vi "LV Mass Compile.vi"   [LabVIEW 2016, in "Script.lvlib"]
uses:
  Script.lvlib
  <vilib>/Wiresmith Technology/G CLI/Argument Parser/Option Class/Option Configuration.ctl
  <vilib>/Wiresmith Technology/G CLI/Argument Parser/Option Class/Argument Type.ctl
  <vilib>/Wiresmith Technology/G CLI/CLI Class/CLI.lvclass
  <vilib>/Wiresmith Technology/G CLI/Argument Parser/Option Class/Option.lvclass
  <vilib>/Wiresmith Technology/G CLI/Argument Parser/Option Set Class/Option Set.lvclass
types:
  T1 = typedef "Option Parser.lvlib/Option.lvclass/Option Configuration.ctl" = cluster{"Option Type":T2, "Option Labels":string[], "Key":string, "Description":string, "Required":bool, "Default Value":string}
  T2 = typedef "Option Parser.lvlib/Option.lvclass/Argument Type.ctl" = enum16{"flag", "value"}
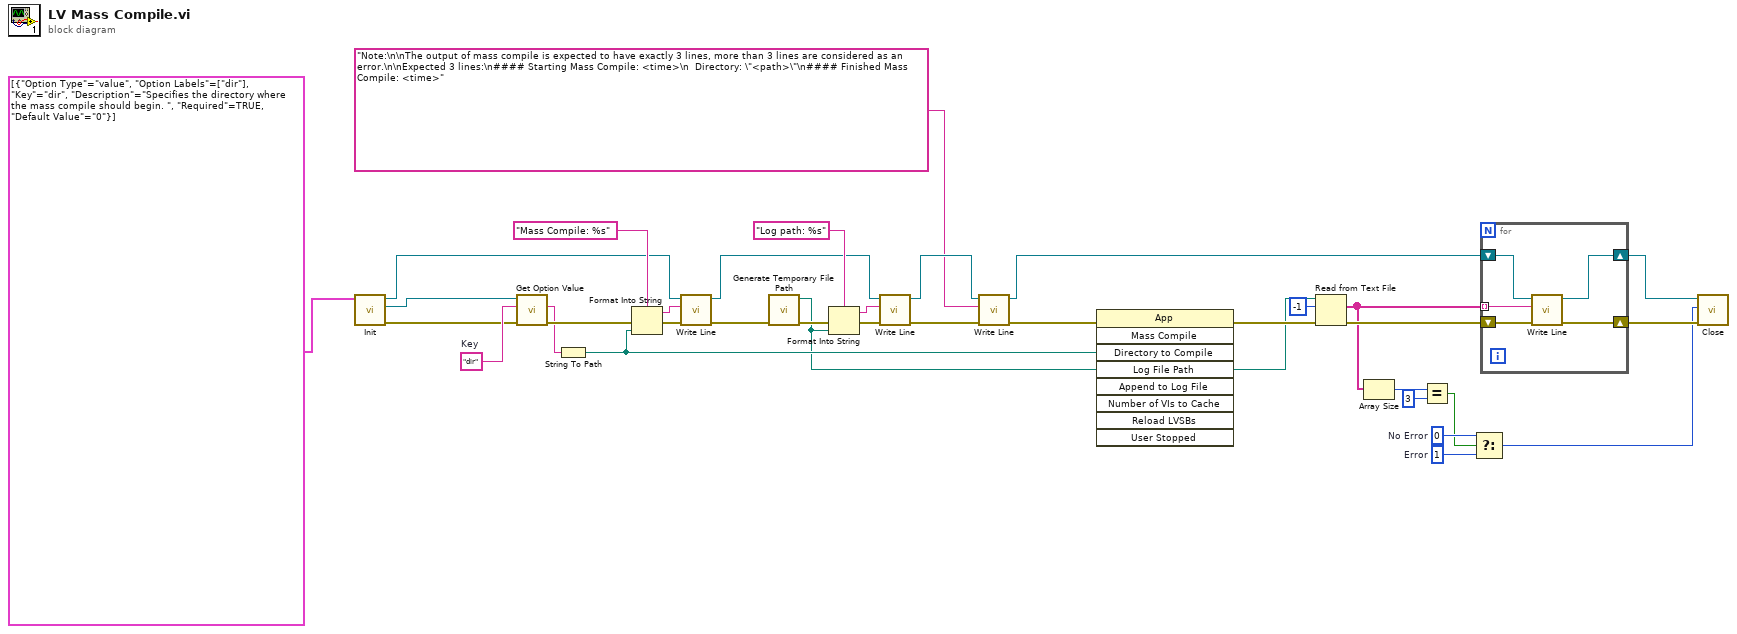
[diagram p0: block diagram]
diagram:
  w10 = 1  # Error
  w11 = 0  # No Error
  w35 = "dir"  # Key
  n1 = call "Init.vi"("Options"=T1[] [{"Option Type"=enum."value", "Option Labels"=["dir"], "Key"="dir", "Description"="Specifies the directory where the mass compile should begin. ", "Required"=TRUE, "Default Value"="0"}]) -> ("error out"=w18:errorcluster, "Option Set out"=w16:refnum<class "Option Set.lvclass">, "CLI out"=w17:refnum<class "CLI.lvclass">)  [unwired: 8 in]
  n2 = call <vilib>:"Get Option Value.vi"("error in (no error)"=w18, "Option Key"=w35, "Option Set in"=w16) -> ("error out"=w30:errorcluster, "Value"=w26:string)  [unwired: 5 in, 2 out]
  n3 = String To Path(string=w26) -> (path=w25:path)
  n4 = Format Into String(format string="Mass Compile: %s", error in=w30, w25) -> (resulting string=w24:string, error out=w29:errorcluster)  [unwired: 1 in]
  n5 = call <vilib>:"Write Line.vi"("error in (no error)"=w29, "Text to Write"=w24, "CLI in"=w17) -> ("error out"=w34:errorcluster, "CLI out"=w27:refnum<class "CLI.lvclass">)  [unwired: 7 in]
  n6 = call <vilib>:"Generate Temporary File Path.vi"("error in (no error)"=w34) -> ("error out"=w33:errorcluster, "Unique Temporary File Path"=w21:path)  [unwired: 9 in]
  n7 = Format Into String(format string="Log path: %s", error in=w33, w21) -> (resulting string=w23:string, error out=w32:errorcluster)  [unwired: 1 in]
  n8 = call <vilib>:"Write Line.vi"("error in (no error)"=w32, "Text to Write"=w23, "CLI in"=w27) -> ("error out"=w5:errorcluster, "CLI out"=w3:refnum<class "CLI.lvclass">)  [unwired: 7 in]
  n9 = call <vilib>:"Write Line.vi"("error in (no error)"=w5, "Text to Write"="Note:\n\nThe output of mass compile is expected to have exactly 3 lines, more than 3 lines are considered as an error.\n\nExpected 3 lines:\n#### Starting Mass Compile: <time>\n  Directory: \"<path>\"\n#### Finished Mass Compile: <time>", "CLI in"=w3) -> ("error out"=w4:errorcluster, "CLI out"=w2:refnum<class "CLI.lvclass">)  [unwired: 7 in]
  n10 = invoke class="App" method="Mass Compile"(error in=w4, "Directory to Compile"=w25, "Log File Path"=w21) -> (error out=w22:errorcluster)  [unwired: 6 in, 8 out]
  n11 = Read from Text File(file (use dialog)=w21, count=-1, error in=w22) -> (text=w9:string[], error out=w19:errorcluster)  [unwired: 1 in, 2 out]
  n12 = Array Size(array=w9) -> (size(s)=w8:i32)
  n13 = Equal?(x=w8, y=3) -> (x = y?=w6:bool)
  n14 = Select(t=w11, s=w6, f=w10) -> (s? t:f=w12:i32)
  n15 = for {
    shift-right: [w37] -> w13
    shift-left: w2 -> [w40]
    shift-right: [w38] -> w14
    shift-left: w19 -> [w39]
    tunnel: w9 -> [w36] mode=indexing
    n16 = call <vilib>:"Write Line.vi"("error in (no error)"=w39, "Text to Write"=w36, "CLI in"=w40) -> ("error out"=w38:errorcluster, "CLI out"=w37:refnum<class "CLI.lvclass">)  [unwired: 7 in]
  }
  n17 = call "Close.vi"("error in (no error)"=w14, "Exit Code (0)"=w12, "CLI in"=w13) -> ()  [unwired: 9 in]
